vi "Lookup Cache Item.vi"(8 "error in (no error)":errorcluster, 10 "ID":string, 11 "Caching in":refnum<class "Caching.lvclass">) -> (0 "error out":errorcluster, 1 "Found?":bool, 2 "Cache Item":T1, 3 "Caching out":refnum<class "Caching.lvclass">)   [LabVIEW 2020, in "HTTP Server.lvlib" / "Caching.lvclass"]
uses:
  Caching.lvclass
  Caching.lvclass/Caching.ctl
  Cache Item.ctl
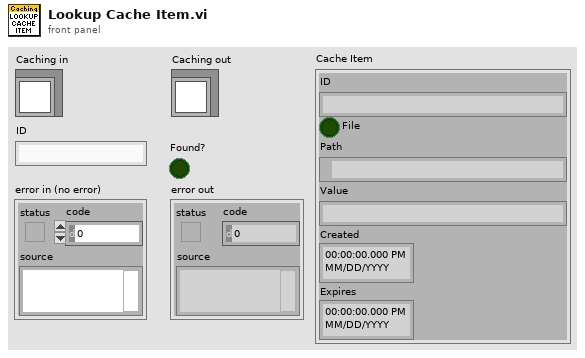
[diagram p1: front panel]
types:
  T1 = typedef "HTTP Server.lvlib/Caching.lvclass/Cache Item.ctl" = cluster{"ID":string, "File":bool, "Path":path, "Value":string, "Created":timestamp, "Expires":timestamp}
  T2 = typedef "HTTP Server.lvlib/Caching.lvclass/Memory Cache.ctl" = cluster{"Size":i64, "Map":map{string, T1}}
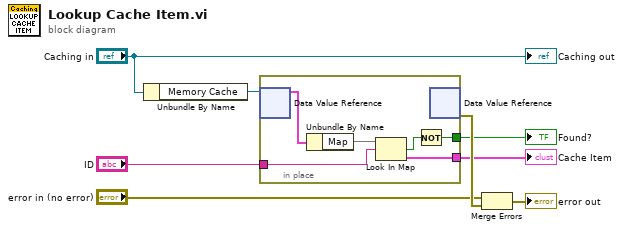
[diagram p0: block diagram]
diagram:
  n1 = Unbundle By Name("Caching in") -> ("Memory Cache"=w6:refnum<data-value>)
  n2 = in-place {
    in-place-border: "ID" -> [w12]
    in-place-border: [w11] -> w4
    in-place-border: [w9] -> w3
    n3 = in-place-dvr #1(w6) -> (w14:T2)  [unwired: 1 out]
    n4 = Unbundle By Name(w14) -> ("Map"=w13:map{string, T1})
    n5 = Look In Map(map=w13, key=w12) -> (key not found?=w10:bool, value=w11:T1)  [unwired: 1 in]
    n6 = Not(x=w10) -> (.not. x?=w9:bool)
    n7 = in-place-dvr #1() -> (w8:errorcluster)  [unwired: 1 in, 1 out]
  }
  "Cache Item" <- w4
  "Found?" <- w3
  n8 = Merge Errors("error in (no error)", w8) -> (→"error out":errorcluster)
  "Caching out" <- "Caching in"
